vi "JeromeErr.vi"(8 "Errin":errorcluster, 9 "CodeERR":string, 10 "RequetteSQL":string, 11 "RetourSQL":string[](array[string])) -> ()   [LabVIEW 2020]
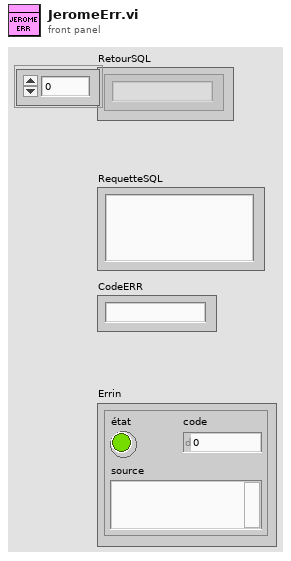
[diagram p1: front panel]
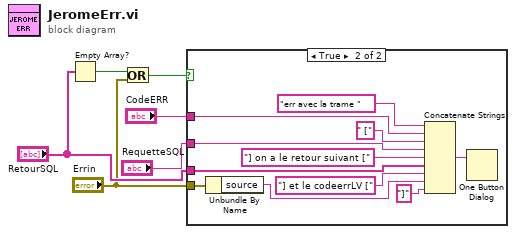
[diagram p0: block diagram]
diagram:
  n1 = Empty Array?(array="RetourSQL") -> (empty?=w2:bool)
  n2 = Or(x=w2, y="Errin") -> (x .or. y?=w3:bool)
  n3 = case shown="True" w3 {
    tunnel: "RequetteSQL" -> [_ w15]
    tunnel: "RetourSQL" -> [_ w13]
    tunnel: "Errin" -> [_ w11]
    tunnel: "CodeERR" -> [_ w7]
    frame False {
    }
    frame True {
      n4 = Unbundle By Name(w11) -> ("source"=w10:string)
      n5 = Concatenate Strings("err avec la trame " ("chaîne"), w7, " [" ("chaîne"), w15, "] on a le retour suivant [" ("chaîne"), w13, "] et le codeerrLV [" ("chaîne"), w10, "]" ("chaîne")) -> (w17:string)
      n6 = One Button Dialog(message=w17) -> ()  [unwired: 1 in, 1 out]
    }
  }
